vi "AB_Engine_Check_Excluded_Directories.vi"(8 "error in (no error)":errorcluster, 10 "Path":path, 11 "directories of excluded files":path[](array[path])) -> (0 "error out":errorcluster, 2 "excluded?":bool)   [LabVIEW 2020]
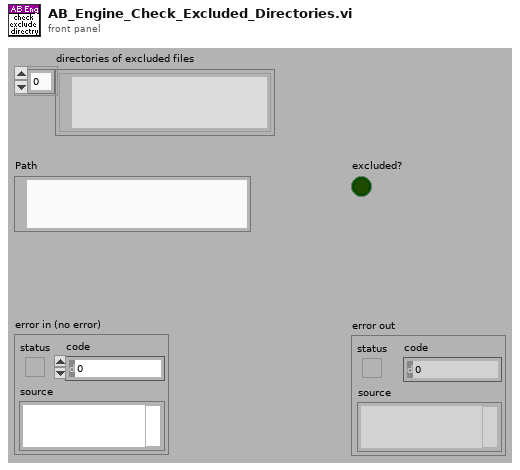
[diagram p1: front panel]
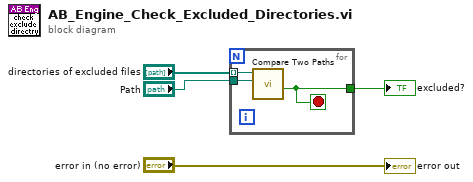
[diagram p0: block diagram]
diagram:
  n1 = for {
    tunnel: "directories of excluded files" -> [w7] mode=indexing
    tunnel: "Path" -> [w6]
    tunnel: [w5] -> w1
    stop <- w5 stop-if-true
    n2 = call <vilib>:"Compare Two Paths.vi"("Path 2"=w6, "Path 1"=w7) -> ("Path 2 Relative to Path 1?"=w5:bool)  [unwired: 6 in, 3 out]
  }
  "excluded?" <- w1
  "error out" <- "error in (no error)"
